vi "Check-selected-filter-types.vi"(7 "Passed? in":bool, 8 "error in":errorcluster, 11 "Data ref in":refnum<data-value>) -> (0 "error IO":errorcluster, 3 "Data ref":refnum<data-value>, 5 "Passed?":bool)   [LabVIEW 2013, in "CameraVision.lvlib" / "CV-Main.lvclass"]
doc: "This function checks if any active filter (monitored or reported) has its corresponding characteristic calculated. An error message is displayed if an active filter characteristic is not calculated.\n\nThis function also updates the temporary filter array with the active filters and collects the header labels for the report file."
uses:
  CV-Main.lvclass
  UI/Popup-messages.ctl
  CV-Main.lvclass/CV-Main.ctl
  Read Filter params.vi
  Read Analysis params.vi
  Read Temperature params.vi
  Filter/CV-Filter.lvclass
  Analysis/CV-Analysis.lvclass
  Temperature/CV-Temperature.lvclass
  UI/CV-UI.lvclass
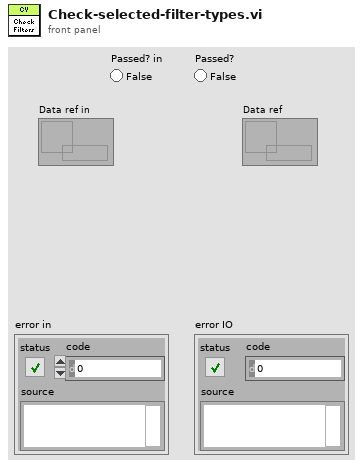
[diagram p1: front panel]
types:
  T1 = typedef "CameraVision.lvlib/CV-UI.lvclass/Popup-messages.ctl" = enum16{"Error-Black image", "Error-Camera config file", "Error-Camera connect", "Error-Grabber init", "Error-Camera setting", "Error-Image offset", "Error-Image import", "Error-Settings file not exist", "Error-Timing source", "Conflict-Filters", "Conflict-Map", "Conflict-Framerate", "Conflict-Charact", "Conflict-Temperature field", "Conflict-Temperature value", "Conflict-Storage-Binary image", "Conflict-Storage-Corrected image", "Conflict-Storage-Map", "Conflict-Storage-Charact", "Conflict-Storage-Temperature field", "Conflict-Storage-Temperature value", "Warning-File exist", "Warning-Parameter reset", "Warning-User cancel", "Info-Images imported"}
  T2 = typedef "CameraVision.lvlib/CV-Filter.lvclass/Filter-characteristic.ctl" = enum16{"Average intensity [0-255]", "Peak intensity [0-255]", "Melt-pool size [mm²]", "Melt-pool aspect ratio []", "Melt-pool fragments []", "Melt-pool position X [pixel]", "Melt-pool position Y [pixel]", "Average temperature [°C]", "Max. temperature [°C]", "Min. temperature [°C]", "Std. dev. temperature [°C]"}
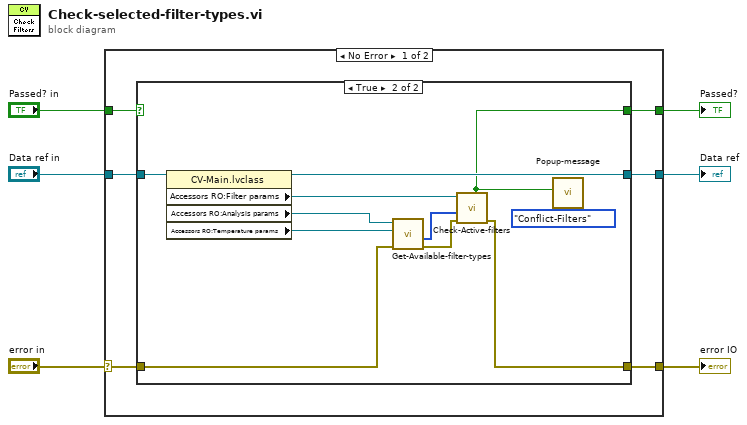
[diagram p0: block diagram]
diagram:
  n1 = case shown="No Error" "error in" {
    selector: "error in" -> [w12 w29]
    tunnel: [w11 w29] -> w5
    tunnel: "Data ref in" -> [w9 w28]
    tunnel: [w10 w28] -> w3
    tunnel: "Passed? in" -> [w8 w27]
    tunnel: [w7 w27] -> w1
    frame No Error {
      n2 = case shown="True" w8 {
        selector: w8 -> [w15 _]
        tunnel: w12 -> [w13 w26]
        tunnel: [w13 w18] -> w11
        tunnel: [w14 w20] -> w10
        tunnel: w9 -> [w14 w21]
        tunnel: [w15 w17] -> w7
        frame False {
        }
        frame True {
          n3 = property class="CV-Main.lvclass"(reference=w21) -> (reference out=w20:refnum<data-value>, "Accessors RO:Filter params"=w25:refnum<data-value>, "Accessors RO:Analysis params"=w24:refnum<data-value>, "Accessors RO:Temperature params"=w23:refnum<data-value>)  [unwired: 1 in, 1 out]
          n4 = call "Get-Available-filter-types.vi"("error in"=w26, "Temp. params. ref."=w23, "Analysis params. ref."=w24) -> ("error IO"=w22:errorcluster, "Available filters"=w19:T2[])  [unwired: 7 in]
          n5 = call "Check-Active-filters.vi"("error in"=w22, "Available filters"=w19, "Filter params. ref. in"=w25) -> ("error IO"=w18:errorcluster, "Passed?"=w17:bool)  [unwired: 6 in, 1 out]
          n6 = call "Popup-message.vi"("Message"=Popup-messages."Conflict-Filters", "Ignore?"=w17) -> ()  [unwired: 9 in, 1 out]
        }
      }
    }
    frame Error {
    }
  }
  "error IO" <- w5
  "Data ref" <- w3
  "Passed?" <- w1
